vi "Calculate Linear Temperature Change.vi"(7 "Ramp Rate deg C/s":dbl=0.05 format="%#_13g", 9 "Time Interval (s)":dbl, 10 "Actual Temperature in":dbl, 11 "Required Temperature deg C":dbl) -> (3 "Actual Temperature out":dbl)   [LabVIEW 2015, in "Thermal Chamber Response Simulator.lvlib"]
doc: "Calculate the temperature change based on the ramp rate and time interval.\n____\nDelacor QMH Thermal Chamber Examples 4.0.0.21\nCopyright (c) 2018, Delacor"
uses:
  Thermal Chamber Response Simulator.lvlib
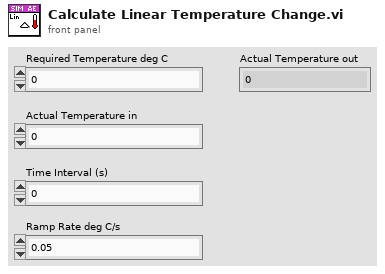
[diagram p1: front panel]
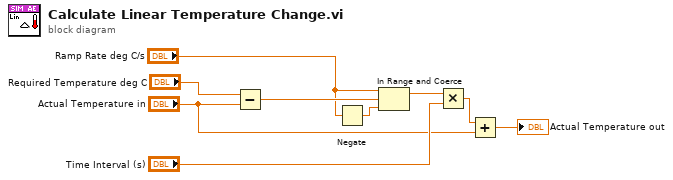
[diagram p0: block diagram]
diagram:
  n1 = Subtract(x="Required Temperature deg C", y="Actual Temperature in") -> (x-y=w3:dbl)
  n2 = Negate(x="Ramp Rate deg C/s") -> (-x=w2:dbl)
  n3 = In Range and Coerce(upper limit="Ramp Rate deg C/s", x=w3, lower limit=w2) -> (coerced(x)=w7:dbl)  [unwired: 1 out]
  n4 = Multiply(x=w7, y="Time Interval (s)") -> (x*y=w8:dbl)
  n5 = Add(x=w8, y="Actual Temperature in") -> (x+y=→"Actual Temperature out":dbl)
